vi "JGE2.vi"() -> ()   [LabVIEW 2019]
doc: "This vi produces a pulse width modulation and you can find power output at various points in time"
panel:
  out "Time array":i32[](array[numeric])=[0, 51, 102, 153, 204, 255, 306, 357, 408, 459, 510, 561, 612, 663, 714, 765, 816, 867, 918, 969, 1020, 1071, 1122, 1173, 1224, 1275, 1326, 1377, 1428, 1479, 1530, 1581, 1632, 1683, 1734, 1785, 1836, 1887, 1938, 1989, 2040, 2091, 2142, 2193, 2244, 2295, 2346, 2397, 2448, 2499, 2550]
  out "Boolean":bool
  out "PW OUT":dbl=1577.843137254902
  in  "Time input":dbl=1750.0
  in  "Timing control":i32=51
  out "?":cluster{"Array":i32[], dbl[]}(graph)={"Array"=[0, 51, 102, 153, 204, 255, 306, 357, 408, 459, 510, 561, 612, 663, 714, 765, 816, 867, 918, 969, 1020, 1071, 1122, 1173, 1224, 1275, 1326, 1377, 1428, 1479, 1530, 1581, 1632, 1683, 1734, 1785, 1836, 1887, 1938, 1989, 2040, 2091, 2142, 2193, 2244, 2295, 2346, 2397, 2448, 2499, 2550], [1050.0, 1083.65, 1117.3, 1150.95, 1184.6, 1218.25, 1251.9, 1285.55, 1319.2, 1352.85, 1386.5, 1420.15, 1453.8, 1487.45, 1521.1, 1554.75, 1588.4, 1622.05, 1655.6999999999998, 1689.35, 1723.0, 1723.0, 1723.0, 1723.0, 1723.0, 1723.0, 1723.0, 1723.0, 1723.0, 1723.0, 1723.0, 1689.35, 1655.6999999999998, 1622.05, 1588.4, 1554.75, 1521.1, 1487.45, 1453.8, 1420.15, 1386.5, 1352.85, 1319.2, 1285.55, 1251.9, 1218.25, 1184.6, 1150.95, 1117.3, 1083.65, 1050.0]}
  out "ramp step":dbl=33.65
  in  "stop":bool
  out "N points":i32=51
  out "PWM array":dbl[](array[numeric])=[1050.0, 1083.65, 1117.3, 1150.95, 1184.6, 1218.25, 1251.9, 1285.55, 1319.2, 1352.85, 1386.5, 1420.15, 1453.8, 1487.45, 1521.1, 1554.75, 1588.4, 1622.05, 1655.6999999999998, 1689.35, 1723.0, 1723.0, 1723.0, 1723.0, 1723.0, 1723.0, 1723.0, 1723.0, 1723.0, 1723.0, 1723.0, 1689.35, 1655.6999999999998, 1622.05, 1588.4, 1554.75, 1521.1, 1487.45, 1453.8, 1420.15, 1386.5, 1352.85, 1319.2, 1285.55, 1251.9, 1218.25, 1184.6, 1150.95, 1117.3, 1083.65, 1050.0]
  in  "N intervals hold":i32=10
  in  "N intervals ramp":i32=20
  in  "hold PW (us)":dbl=1723.0
  in  "start PW (us)":dbl=1050.0
  # "Speed Control"
  # "Time input (s)"
  # "Juan Gamez\nP3600\nEP2"
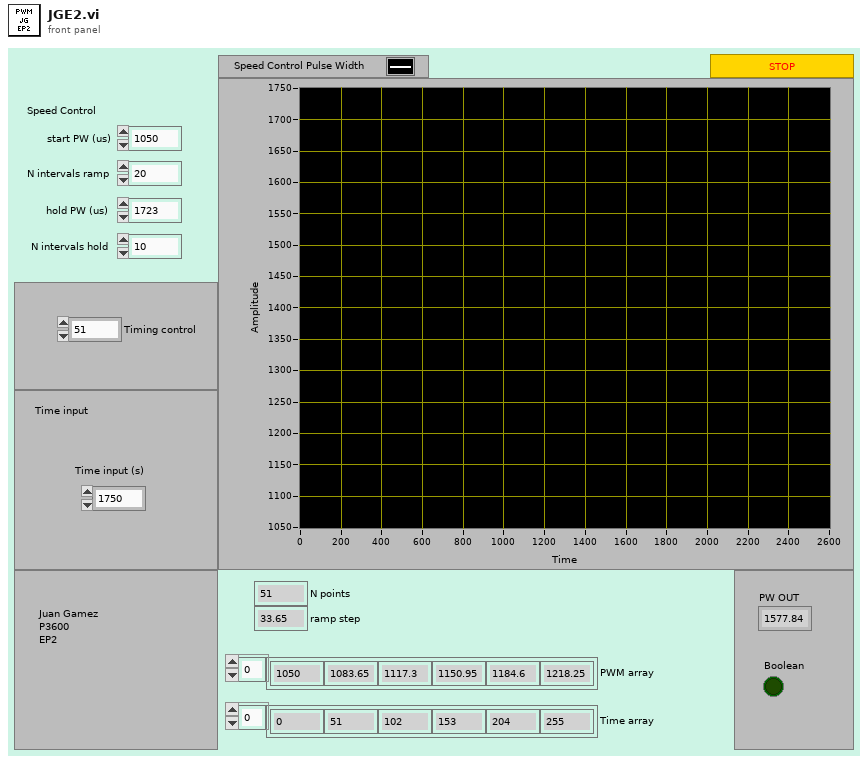
[diagram p1: front panel]
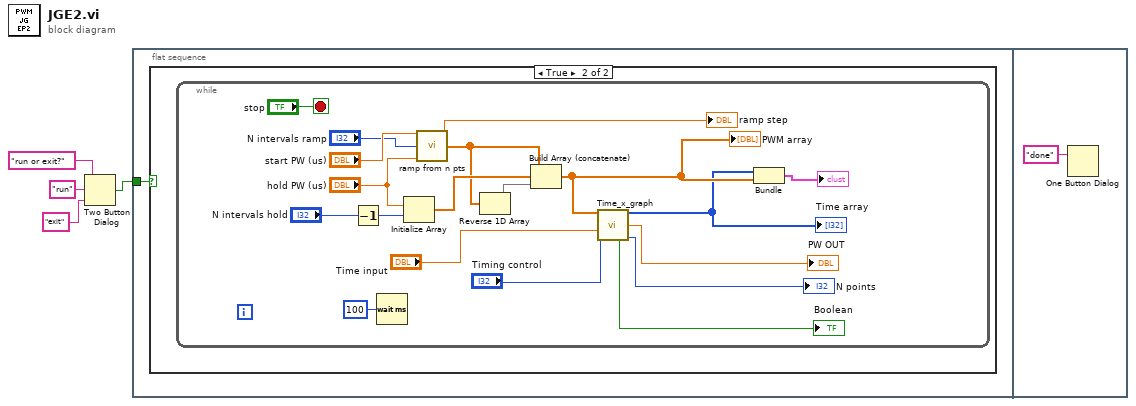
[diagram p0: block diagram]
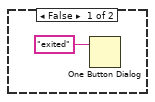
[diagram p2: hidden frame]
diagram:
  n1 = Two Button Dialog(message="run or exit?", 1:"exit" ("F button name (\"Cancel\")"), 2:"run" ("T button name (\"OK\")")) -> (T button?=w1:bool)
  n2 = flat-sequence {
    tunnel: w1 -> [w5]
    frame #0 {
      n3 = case shown="True" w5 {
        frame False {
          n4 = One Button Dialog(message="exited" ("button name (\"OK\")")) -> ()  [unwired: 1 in, 1 out]
        }
        frame True {
          n5 = while {
            stop <- "stop" stop-if-true
            n6 = Decrement(x="N intervals hold") -> (x-1=w15:i32)
            n7 = Wait (ms)(milliseconds to wait=u32 100) -> ()  [unwired: 1 out]
            n8 = Initialize Array("hold PW (us)", w15) -> (w23:dbl[])
            n9 = call "ramp from n pts.vi"("start value"="start PW (us)", "N intervals"="N intervals ramp", "end value"="hold PW (us)") -> ("ramp step"=→"ramp step":dbl, "Values array"=w22:dbl[])  [unwired: 10 in, 1 out]
            n10 = Reverse 1D Array(array=w22) -> (reversed array=w21:dbl[])
            n11 = Build Array (concatenate)(w22, w23, w21) -> (w13:dbl[])
            "PWM array" <- w13
            n12 = call "Time_x_graph.vi"("Inital array"=w13, "Time inputs"="Time input", "Timing control"="Timing control") -> ("Array"=w10:i32[], "PW OUT"=→"PW OUT":dbl, "Boolean 2"=→"Boolean":bool, "N points"=→"N points":i32)  [unwired: 9 in]
            "Time array" <- w10
            n13 = Bundle("Array"=w10, w13) -> (→"?":cluster{"Array":i32[], dbl[]})  [unwired: 1 in]
          }
        }
      }
    }
    frame #1 {
      n14 = One Button Dialog(message="done" ("button name (\"OK\")")) -> ()  [unwired: 1 in, 1 out]
    }
  }
